vi "Set Force Sensor Settings.vi"(10 "Force Sensor Settings":T1={"Reference Voltage Vref"=0.0, "FC1 Force Sensor"={"Capacity"=1.0, "Sensitivity"=0.001}, "FC2 Force Sensor"={"Capacity"=1.0, "Sensitivity"=0.001}} {"FC2 Force Sensor"."Sensitivity" min=0.001 max=5000.0 format="%.4f"; "FC2 Force Sensor"."Capacity" min=1.0 max=5000000.0 format="%.4f"; "FC1 Force Sensor"."Sensitivity" min=0.001 max=5000.0 format="%.4f"; "FC1 Force Sensor"."Capacity" min=1.0 max=5000000.0 format="%.4f"; "Reference Voltage Vref" min=-10.0 max=10.0 format="%.3f"}, 11 "Model in":refnum<class "Model.lvclass">) -> (3 "Model out":refnum<class "Model.lvclass">)   [LabVIEW 2015, in "Model.lvclass"]
uses:
  Model.lvclass
  Typedefs/Force Sensor Settings.ctl
  <userlib>/Common/Devices/ForceSensorCalculator/Config/ForceSensorCalculator.ctl
  Model.lvclass/Model.ctl
  Typedefs/FAMT Typedefs.lvlib
  <userlib>/Common/Devices/ForceSensorCalculator/ForceSensorCalculator.lvlib
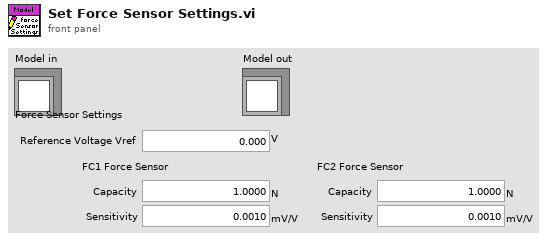
[diagram p1: front panel]
types:
  T1 = typedef "FAMT Typedefs.lvlib/Force Sensor Settings.ctl" = cluster{"Reference Voltage Vref":dbl[unit], "FC1 Force Sensor":T2, "FC2 Force Sensor":T2}
  T2 = typedef "ForceSensorCalculator.lvlib/ForceSensorCalculator.ctl" = cluster{"Capacity":dbl[unit], "Sensitivity":dbl[unit]}
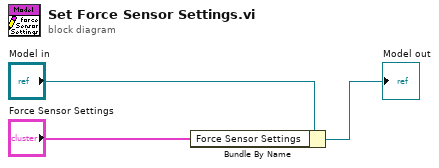
[diagram p0: block diagram]
diagram:
  n1 = Bundle By Name(cluster="Model in", "Force Sensor Settings"="Force Sensor Settings") -> (→"Model out":refnum<class "Model.lvclass">)
